vi "Pndt byte splitter - U32.vi"(9 "byte U32":u32 format="%.0b", 10 "mask size":u32, 11 "shift right":i16) -> (1 "lo":u32 format="%.0b", 3 "hi":u32 format="%.0b")   [LabVIEW 2026, in "MicroPulse_Driver.lvlib"]
uses:
  MicroPulse_Driver.lvlib
panel:
  # "msb"
  # "lsb"
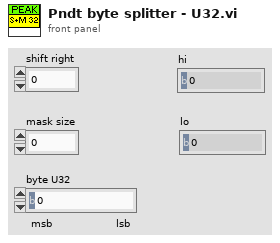
[diagram p1: front panel]
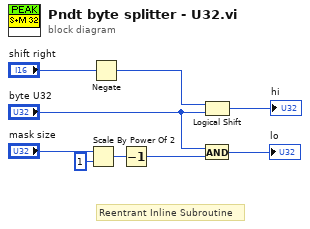
[diagram p0: block diagram]
diagram:
  # "Reentrant Inline Subroutine"
  n1 = Scale By Power Of 2(n="mask size", x=u32 1) -> (x*2^n=w2:u32)
  n2 = Negate(x="shift right") -> (-x=w8:i16)
  n3 = Decrement(x=w2) -> (x-1=w1:u32)
  n4 = Logical Shift(y=w8, x="byte U32") -> (x << y=→"hi":u32)
  n5 = And(x="byte U32", y=w1) -> (x .and. y?=→"lo":u32)
